vi "Serialize - JSON.vi"(8 "error in":errorcluster, 11 "PAS Data in":refnum<class "PAS Data.lvclass">) -> (0 "error out":errorcluster, 2 "Serialized JSON":string, 3 "PAS Data out":refnum<class "PAS Data.lvclass">)   [LabVIEW 2014, in "PAS Library.lvlib" / "PAS Data.lvclass"]
uses:
  PAS Data.lvclass
  PAS Data.lvclass/PAS Data.ctl
  Cell/PAS Cell Data.lvclass
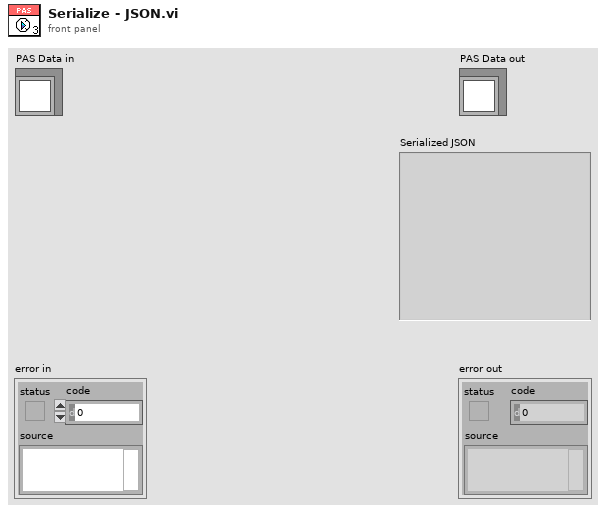
[diagram p1: front panel]
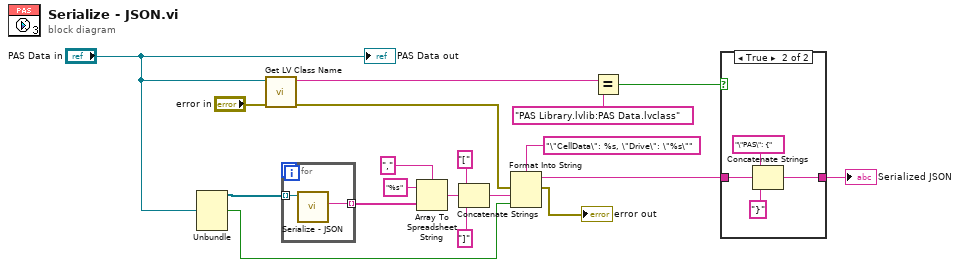
[diagram p0: block diagram]
diagram:
  n1 = Unbundle("PAS Data in") -> (w19:refnum<class "PAS Cell Data.lvclass">[], w10:bool)  [unwired: 3 out]
  n2 = call <vilib>:"Get LV Class Name.vi"("error in (no error)"="error in", "object"="PAS Data in") -> ("error out"=w2:errorcluster, "class name"=w8:string)  [unwired: 8 in]
  n3 = for {
    tunnel: w19 -> [w21] mode=indexing
    tunnel: [w20] -> w18 mode=indexing
    n4 = call-dynamic "Serialize - JSON.vi"("PAS Cell Data in"=w21) -> ("Serialized JSON"=w20:string)  [unwired: 8 in, 2 out]
  }
  n5 = Array To Spreadsheet String(delimiter (Tab)=",", array=w18, 3:"%s" ("format string")) -> (spreadsheet string=w15:string)
  n6 = Concatenate Strings("[" ("string"), w15, "]" ("string")) -> (w12:string)
  n7 = Format Into String(format string="\"CellData\": %s, \"Drive\": \"%s\"", error in=w2, w12, w10) -> (resulting string=w5:string, error out=→"error out":errorcluster)  [unwired: 1 in]
  n8 = Equal?(x=w8, y="PAS Library.lvlib:PAS Data.lvclass") -> (x = y?=w6:bool)
  n9 = case shown="True" w6 {
    tunnel: w5 -> [w22 w26]
    tunnel: [w22 w23] -> w4
    frame False {
    }
    frame True {
      n10 = Concatenate Strings("\"PAS\": {" ("string"), w26, "}" ("string")) -> (w23:string)
    }
  }
  "Serialized JSON" <- w4
  "PAS Data out" <- "PAS Data in"
